vi "Start Module.vi"(8 "error in (no error)":errorcluster, 11 "Module in":refnum<class "Module.lvclass">) -> (0 "error out":errorcluster, 3 "Module out":refnum<class "Module.lvclass">)   [LabVIEW 2020, in "Volatus.lvlib" / "Module.lvclass"]
uses:
  Module.lvclass
  State.ctl
  Module Identity/Module Identity.lvclass/Module Identity.ctl
  Module.lvclass/Module.ctl
  Module Identity/Module Identity.lvclass
  C:/dev/lv20CE/relink/lv-volatus/Volatus/Identity/Identity.lvclass
  VolatusAPI/VolatusAPI.lvclass
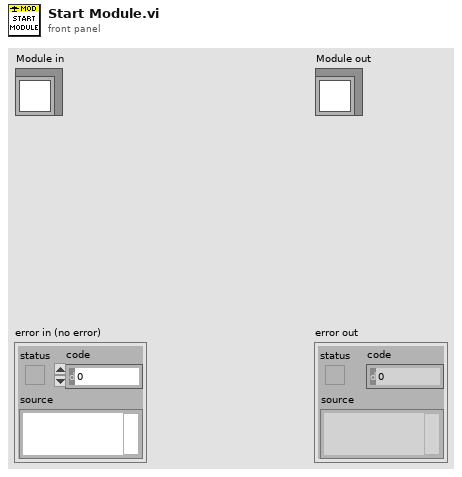
[diagram p1: front panel]
types:
  T1 = typedef "Volatus.lvlib/Module.lvclass/State.ctl" = enum16{"Unknown", "Launched", "Starting", "Running", "Stopping", "Stopped", "Error - Starting", "Error - Run", "Error - Stopping"}
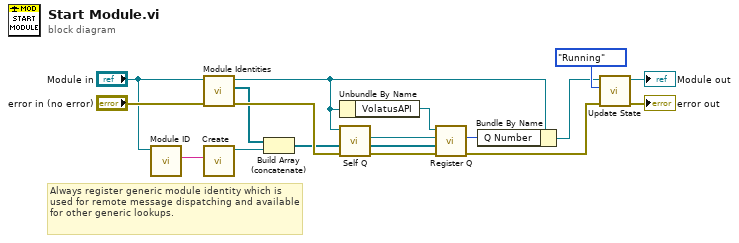
[diagram p0: block diagram]
diagram:
  # "Always register generic module identity which is used for remote message dispatching and available for other generic lookups."
  n1 = call-dynamic "Module ID.vi"("Module in"="Module in") -> ("Module ID"=w2:string)  [unwired: 10 in]
  n2 = call-dynamic "Module Identities.vi"("error in (no error)"="error in (no error)", "Module in"="Module in") -> ("error out"=w12:errorcluster, "Identities"=w8:refnum<class "Identity.lvclass">[], "Module out"=w11:refnum<class "Module.lvclass">)  [unwired: 7 in]
  n3 = call "Create.vi"("ID"=w2) -> ("Module Identity out"=w3:refnum<class "Module Identity.lvclass">)  [unwired: 10 in]
  n4 = Build Array (concatenate)(w8, w3) -> (w4:refnum<class "Identity.lvclass">[])
  n5 = Unbundle By Name(w11) -> ("VolatusAPI"=w7:refnum<class "VolatusAPI.lvclass">)
  n6 = call "Self Q.vi"("Module in"=w11) -> ("Self Q"=w6:refnum<class "MessageQ.lvclass">)  [unwired: 9 in, 1 out]
  n7 = call "Register Q.vi"("error in (no error)"=w12, "Identities"=w4, "MessageQ"=w6, "VolatusAPI in"=w7) -> ("error out"=w9:errorcluster, "Q Number"=w5:i32)  [unwired: 5 in, 1 out]
  n8 = Bundle By Name(cluster=w11, "Q Number"=w5) -> (w10:refnum<class "Module.lvclass">)
  n9 = call "Update State.vi"("error in (no error)"=w9, "State"=State."Running" ("f"), "Module in"=w10) -> ("error out"=→"error out":errorcluster, "Module out"=→"Module out":refnum<class "Module.lvclass">)  [unwired: 7 in]
